vi "Create Database For Box IDs from cluster.vi"(8 "error in (no error)":errorcluster, 10 "Box ID Array":u8[](array[numeric])=[1, 2, 3, 4, 5, 6, 7, 8, 9, 10, 11, 12, 13, 14, 15], 11 "Calibration mode":bool) -> (0 "error out":errorcluster, 2 "Specific Frames":refnum<k21>[](array[refnum]), 3 "XNET Database out":refnum<k21>)   [LabVIEW 2021, in "BS120x Driver.lvlib" / "BS120x.lvclass"]
uses:
  BS120x.lvclass
  XNET Signal properties.ctl
  XNET Frame properties.ctl
  <vilib>/xnet/xnet.llb/XNET Database Create (Cluster).vi
  <vilib>/xnet/xnet.llb/XNET Database Create (Frame).vi
  <vilib>/xnet/xnet.llb/XNET Database Create (Signal).vi
  <resource>/objmgr/xnet.rc
panel:
  in  "Frames (Standard)":cluster{T1[], "XNET Frame properties":T2}[](array[cluster])=[{[{"ByteOrdr"=0, "Comment"="", "DataType"=1, "Default"=0.0, "Max"=5.0, "Min"=0.0, "NameShort"="AI_1", "NumBits"=16, "ScaleFac"=0.0001, "ScaleOff"=0.0, "StartBit"=0, "Unit"="V"}, {"ByteOrdr"=0, "Comment"="", "DataType"=1, "Default"=0.0, "Max"=5.0, "Min"=0.0, "NameShort"="AI_2", "NumBits"=16, "ScaleFac"=0.0001, "ScaleOff"=0.0, "StartBit"=16, "Unit"="V"}, {"ByteOrdr"=0, "Comment"="", "DataType"=1, "Default"=0.0, "Max"=5.0, "Min"=0.0, "NameShort"="AI_3", "NumBits"=16, "ScaleFac"=0.0001, "ScaleOff"=0.0, "StartBit"=32, "Unit"="V"}, {"ByteOrdr"=0, "Comment"="", "DataType"=1, "Default"=0.0, "Max"=5.0, "Min"=0.0, "NameShort"="AI_4", "NumBits"=16, "ScaleFac"=0.0001, "ScaleOff"=0.0, "StartBit"=48, "Unit"="V"}], "XNET Frame properties"={"NameShort"="AI_Readback_1_4", "ID"=672, "PayldLen"=8, "CAN.TimingType"=0, "CAN.TxTime"=0.01}}, {[{"ByteOrdr"=0, "Comment"="", "DataType"=1, "Default"=0.0, "Max"=5.0, "Min"=0.0, "NameShort"="AI_5", "NumBits"=16, "ScaleFac"=0.0001, "ScaleOff"=0.0, "StartBit"=0, "Unit"="V"}, {"ByteOrdr"=0, "Comment"="", "DataType"=1, "Default"=0.0, "Max"=5.0, "Min"=0.0, "NameShort"="AI_6", "NumBits"=16, "ScaleFac"=0.0001, "ScaleOff"=0.0, "StartBit"=16, "Unit"="V"}, {"ByteOrdr"=0, "Comment"="", "DataType"=1, "Default"=0.0, "Max"=5.0, "Min"=0.0, "NameShort"="AI_7", "NumBits"=16, "ScaleFac"=0.0001, "ScaleOff"=0.0, "StartBit"=32, "Unit"="V"}, {"ByteOrdr"=0, "Comment"="", "DataType"=1, "Default"=0.0, "Max"=5.0, "Min"=0.0, "NameShort"="AI_8", "NumBits"=16, "ScaleFac"=0.0001, "ScaleOff"=0.0, "StartBit"=48, "Unit"="V"}], "XNET Frame properties"={"NameShort"="AI_Readback_5_8", "ID"=688, "PayldLen"=8, "CAN.TimingType"=0, "CAN.TxTime"=0.01}}, {[{"ByteOrdr"=0, "Comment"="", "DataType"=1, "Default"=0.0, "Max"=5.0, "Min"=0.0, "NameShort"="AO1_Voltage", "NumBits"=16, "ScaleFac"=0.0001, "ScaleOff"=0.0, "StartBit"=0, "Unit"="V"}, {"ByteOrdr"=0, "Comment"="", "DataType"=1, "Default"=0.0, "Max"=5.0, "Min"=0.0, "NameShort"="AO2_Voltage", "NumBits"=16, "ScaleFac"=0.0001, "ScaleOff"=0.0, "StartBit"=16, "Unit"="V"}], "XNET Frame properties"={"NameShort"="Analog_Out_Set_1_2", "ID"=544, "PayldLen"=8, "CAN.TimingType"=1, "CAN.TxTime"=0.1}}, {[{"ByteOrdr"=0, "Comment"="", "DataType"=1, "Default"=1.0, "Max"=12.0, "Min"=1.0, "NameShort"="Channel", "NumBits"=8, "ScaleFac"=1.0, "ScaleOff"=1.0, "StartBit"=0, "Unit"=""}, {"ByteOrdr"=0, "Comment"="", "DataType"=1, "Default"=0.0, "Max"=1.0, "Min"=0.0, "NameShort"="Enable", "NumBits"=1, "ScaleFac"=1.0, "ScaleOff"=0.0, "StartBit"=8, "Unit"=""}], "XNET Frame properties"={"NameShort"="Cell_Enable", "ID"=1360, "PayldLen"=2, "CAN.TimingType"=1, "CAN.TxTime"=0.1}}, {[{"ByteOrdr"=0, "Comment"="", "DataType"=1, "Default"=0.0, "Max"=1.0, "Min"=0.0, "NameShort"="Enable", "NumBits"=1, "ScaleFac"=1.0, "ScaleOff"=0.0, "StartBit"=0, "Unit"=""}], "XNET Frame properties"={"NameShort"="Cell_Enable_All", "ID"=1344, "PayldLen"=1, "CAN.TimingType"=1, "CAN.TxTime"=0.1}}, {[{"ByteOrdr"=0, "Comment"="", "DataType"=1, "Default"=0.0, "Max"=500.0000000000003, "Min"=-500.0000000000003, "NameShort"="Cell_I_1", "NumBits"=16, "ScaleFac"=0.1, "ScaleOff"=-3276.800000000003, "StartBit"=0, "Unit"="mA"}, {"ByteOrdr"=0, "Comment"="", "DataType"=1, "Default"=0.0, "Max"=500.0000000000003, "Min"=-500.0000000000003, "NameShort"="Cell_I_2", "NumBits"=16, "ScaleFac"=0.1, "ScaleOff"=-3276.800000000003, "StartBit"=16, "Unit"="mA"}, {"ByteOrdr"=0, "Comment"="", "DataType"=1, "Default"=0.0, "Max"=500.0000000000003, "Min"=-500.0000000000003, "NameShort"="Cell_I_3", "NumBits"=16, "ScaleFac"=0.1, "ScaleOff"=-3276.800000000003, "StartBit"=32, "Unit"="mA"}, {"ByteOrdr"=0, "Comment"="", "DataType"=1, "Default"=0.0, "Max"=500.0000000000003, "Min"=-500.0000000000003, "NameShort"="Cell_I_4", "NumBits"=16, "ScaleFac"=0.1, "ScaleOff"=-3276.800000000003, "StartBit"=48, "Unit"="mA"}], "XNET Frame properties"={"NameShort"="Cell_I_Readback_1_4", "ID"=384, "PayldLen"=8, "CAN.TimingType"=0, "CAN.TxTime"=0.01}}, {[{"ByteOrdr"=0, "Comment"="", "DataType"=1, "Default"=0.0, "Max"=500.0000000000003, "Min"=-500.0000000000003, "NameShort"="Cell_I_5", "NumBits"=16, "ScaleFac"=0.1, "ScaleOff"=-3276.800000000003, "StartBit"=0, "Unit"="mA"}, {"ByteOrdr"=0, "Comment"="", "DataType"=1, "Default"=0.0, "Max"=500.0000000000003, "Min"=-500.0000000000003, "NameShort"="Cell_I_6", "NumBits"=16, "ScaleFac"=0.1, "ScaleOff"=-3276.800000000003, "StartBit"=16, "Unit"="mA"}, {"ByteOrdr"=0, "Comment"="", "DataType"=1, "Default"=0.0, "Max"=500.0000000000003, "Min"=-500.0000000000003, "NameShort"="Cell_I_7", "NumBits"=16, "ScaleFac"=0.1, "ScaleOff"=-3276.800000000003, "StartBit"=32, "Unit"="mA"}, {"ByteOrdr"=0, "Comment"="", "DataType"=1, "Default"=0.0, "Max"=500.0000000000003, "Min"=-500.0000000000003, "NameShort"="Cell_I_8", "NumBits"=16, "ScaleFac"=0.1, "ScaleOff"=-3276.800000000003, "StartBit"=48, "Unit"="mA"}], "XNET Frame properties"={"NameShort"="Cell_I_Readback_5_8", "ID"=400, "PayldLen"=8, "CAN.TimingType"=0, "CAN.TxTime"=0.01}}, {[{"ByteOrdr"=0, "Comment"="", "DataType"=1, "Default"=0.0, "Max"=500.0000000000003, "Min"=-500.0000000000003, "NameShort"="Cell_I_09", "NumBits"=16, "ScaleFac"=0.1, "ScaleOff"=-3276.800000000003, "StartBit"=0, "Unit"="mA"}, {"ByteOrdr"=0, "Comment"="", "DataType"=1, "Default"=0.0, "Max"=500.0000000000003, "Min"=-500.0000000000003, "NameShort"="Cell_I_10", "NumBits"=16, "ScaleFac"=0.1, "ScaleOff"=-3276.800000000003, "StartBit"=16, "Unit"="mA"}, {"ByteOrdr"=0, "Comment"="", "DataType"=1, "Default"=0.0, "Max"=500.0000000000003, "Min"=-500.0000000000003, "NameShort"="Cell_I_11", "NumBits"=16, "ScaleFac"=0.1, "ScaleOff"=-3276.800000000003, "StartBit"=32, "Unit"="mA"}, {"ByteOrdr"=0, "Comment"="", "DataType"=1, "Default"=0.0, "Max"=500.0000000000003, "Min"=-500.0000000000003, "NameShort"="Cell_I_12", "NumBits"=16, "ScaleFac"=0.1, "ScaleOff"=-3276.800000000003, "StartBit"=48, "Unit"="mA"}], "XNET Frame properties"={"NameShort"="Cell_I_Readback_9_12", "ID"=416, "PayldLen"=8, "CAN.TimingType"=0, "CAN.TxTime"=0.01}}, {[{"ByteOrdr"=0, "Comment"="", "DataType"=1, "Default"=0.0, "Max"=500.0000000000003, "Min"=-500.0000000000003, "NameShort"="Sink_I_All", "NumBits"=16, "ScaleFac"=0.1, "ScaleOff"=0.0, "StartBit"=16, "Unit"="mA"}, {"ByteOrdr"=0, "Comment"="", "DataType"=1, "Default"=0.0, "Max"=500.0000000000003, "Min"=-500.0000000000003, "NameShort"="Source_I_All", "NumBits"=16, "ScaleFac"=0.1, "ScaleOff"=0.0, "StartBit"=0, "Unit"="mA"}], "XNET Frame properties"={"NameShort"="Cell_I_Set_All", "ID"=1152, "PayldLen"=4, "CAN.TimingType"=1, "CAN.TxTime"=0.1}}, {[{"ByteOrdr"=0, "Comment"="", "DataType"=1, "Default"=1.0, "Max"=12.0, "Min"=1.0, "NameShort"="Channel", "NumBits"=8, "ScaleFac"=1.0, "ScaleOff"=1.0, "StartBit"=0, "Unit"=""}, {"ByteOrdr"=0, "Comment"="", "DataType"=1, "Default"=0.0, "Max"=500.0000000000003, "Min"=-500.0000000000003, "NameShort"="I_Sink", "NumBits"=16, "ScaleFac"=0.1, "ScaleOff"=0.0, "StartBit"=8, "Unit"="mA"}], "XNET Frame properties"={"NameShort"="Cell_I_Sink_Set", "ID"=1184, "PayldLen"=3, "CAN.TimingType"=1, "CAN.TxTime"=0.1}}, {[{"ByteOrdr"=0, "Comment"="", "DataType"=1, "Default"=1.0, "Max"=12.0, "Min"=1.0, "NameShort"="Channel", "NumBits"=8, "ScaleFac"=1.0, "ScaleOff"=1.0, "StartBit"=0, "Unit"=""}, {"ByteOrdr"=0, "Comment"="", "DataType"=1, "Default"=0.0, "Max"=500.0000000000003, "Min"=-500.0000000000003, "NameShort"="I_Source", "NumBits"=16, "ScaleFac"=0.1, "ScaleOff"=0.0, "StartBit"=8, "Unit"="mA"}], "XNET Frame properties"={"NameShort"="Cell_I_Source_Set", "ID"=1200, "PayldLen"=3, "CAN.TimingType"=1, "CAN.TxTime"=0.1}}, {[{"ByteOrdr"=0, "Comment"="", "DataType"=1, "Default"=0.0, "Max"=5.0, "Min"=0.0, "NameShort"="Cell_V_1", "NumBits"=16, "ScaleFac"=0.0001, "ScaleOff"=0.0, "StartBit"=0, "Unit"="V"}, {"ByteOrdr"=0, "Comment"="", "DataType"=1, "Default"=0.0, "Max"=5.0, "Min"=0.0, "NameShort"="Cell_V_2", "NumBits"=16, "ScaleFac"=0.0001, "ScaleOff"=0.0, "StartBit"=16, "Unit"="V"}, {"ByteOrdr"=0, "Comment"="", "DataType"=1, "Default"=0.0, "Max"=5.0, "Min"=0.0, "NameShort"="Cell_V_3", "NumBits"=16, "ScaleFac"=0.0001, "ScaleOff"=0.0, "StartBit"=32, "Unit"="V"}, {"ByteOrdr"=0, "Comment"="", "DataType"=1, "Default"=0.0, "Max"=5.0, "Min"=0.0, "NameShort"="Cell_V_4", "NumBits"=16, "ScaleFac"=0.0001, "ScaleOff"=0.0, "StartBit"=48, "Unit"="V"}], "XNET Frame properties"={"NameShort"="Cell_V_Readback_1_4", "ID"=288, "PayldLen"=8, "CAN.TimingType"=0, "CAN.TxTime"=0.01}}, {[{"ByteOrdr"=0, "Comment"="", "DataType"=1, "Default"=0.0, "Max"=5.0, "Min"=0.0, "NameShort"="Cell_V_5", "NumBits"=16, "ScaleFac"=0.0001, "ScaleOff"=0.0, "StartBit"=0, "Unit"="V"}, {"ByteOrdr"=0, "Comment"="", "DataType"=1, "Default"=0.0, "Max"=5.0, "Min"=0.0, "NameShort"="Cell_V_6", "NumBits"=16, "ScaleFac"=0.0001, "ScaleOff"=0.0, "StartBit"=16, "Unit"="V"}, {"ByteOrdr"=0, "Comment"="", "DataType"=1, "Default"=0.0, "Max"=5.0, "Min"=0.0, "NameShort"="Cell_V_7", "NumBits"=16, "ScaleFac"=0.0001, "ScaleOff"=0.0, "StartBit"=32, "Unit"="V"}, {"ByteOrdr"=0, "Comment"="", "DataType"=1, "Default"=0.0, "Max"=5.0, "Min"=0.0, "NameShort"="Cell_V_8", "NumBits"=16, "ScaleFac"=0.0001, "ScaleOff"=0.0, "StartBit"=48, "Unit"="V"}], "XNET Frame properties"={"NameShort"="Cell_V_Readback_5_8", "ID"=304, "PayldLen"=8, "CAN.TimingType"=0, "CAN.TxTime"=0.01}}, {[{"ByteOrdr"=0, "Comment"="", "DataType"=1, "Default"=0.0, "Max"=5.0, "Min"=0.0, "NameShort"="Cell_V_09", "NumBits"=16, "ScaleFac"=0.0001, "ScaleOff"=0.0, "StartBit"=0, "Unit"="V"}, {"ByteOrdr"=0, "Comment"="", "DataType"=1, "Default"=0.0, "Max"=5.0, "Min"=0.0, "NameShort"="Cell_V_10", "NumBits"=16, "ScaleFac"=0.0001, "ScaleOff"=0.0, "StartBit"=16, "Unit"="V"}, {"ByteOrdr"=0, "Comment"="", "DataType"=1, "Default"=0.0, "Max"=5.0, "Min"=0.0, "NameShort"="Cell_V_11", "NumBits"=16, "ScaleFac"=0.0001, "ScaleOff"=0.0, "StartBit"=32, "Unit"="V"}, {"ByteOrdr"=0, "Comment"="", "DataType"=1, "Default"=0.0, "Max"=5.0, "Min"=0.0, "NameShort"="Cell_V_12", "NumBits"=16, "ScaleFac"=0.0001, "ScaleOff"=0.0, "StartBit"=48, "Unit"="V"}], "XNET Frame properties"={"NameShort"="Cell_V_Readback_9_12", "ID"=320, "PayldLen"=8, "CAN.TimingType"=0, "CAN.TxTime"=0.01}}, {[{"ByteOrdr"=0, "Comment"="", "DataType"=1, "Default"=0.0, "Max"=5.0, "Min"=0.0, "NameShort"="Cell_Voltage", "NumBits"=16, "ScaleFac"=0.0001, "ScaleOff"=0.0, "StartBit"=8, "Unit"="V"}, {"ByteOrdr"=0, "Comment"="", "DataType"=1, "Default"=1.0, "Max"=12.0, "Min"=1.0, "NameShort"="Channel", "NumBits"=8, "ScaleFac"=1.0, "ScaleOff"=1.0, "StartBit"=0, "Unit"=""}], "XNET Frame properties"={"NameShort"="Cell_V_Set", "ID"=1296, "PayldLen"=3, "CAN.TimingType"=1, "CAN.TxTime"=0.1}}, {[{"ByteOrdr"=0, "Comment"="", "DataType"=1, "Default"=0.0, "Max"=5.0, "Min"=0.0, "NameShort"="Cell_1_Voltage", "NumBits"=16, "ScaleFac"=0.0001, "ScaleOff"=0.0, "StartBit"=0, "Unit"="V"}, {"ByteOrdr"=0, "Comment"="", "DataType"=1, "Default"=0.0, "Max"=5.0, "Min"=0.0, "NameShort"="Cell_2_Voltage", "NumBits"=16, "ScaleFac"=0.0001, "ScaleOff"=0.0, "StartBit"=16, "Unit"="V"}, {"ByteOrdr"=0, "Comment"="", "DataType"=1, "Default"=0.0, "Max"=5.0, "Min"=0.0, "NameShort"="Cell_3_Voltage", "NumBits"=16, "ScaleFac"=0.0001, "ScaleOff"=0.0, "StartBit"=32, "Unit"="V"}, {"ByteOrdr"=0, "Comment"="", "DataType"=1, "Default"=0.0, "Max"=5.0, "Min"=0.0, "NameShort"="Cell_4_Voltage", "NumBits"=16, "ScaleFac"=0.0001, "ScaleOff"=0.0, "StartBit"=48, "Unit"=""}], "XNET Frame properties"={"NameShort"="Cell_V_Set_1_4", "ID"=160, "PayldLen"=8, "CAN.TimingType"=1, "CAN.TxTime"=0.1}}, {[{"ByteOrdr"=0, "Comment"="", "DataType"=1, "Default"=0.0, "Max"=5.0, "Min"=0.0, "NameShort"="Cell_5_Voltage", "NumBits"=16, "ScaleFac"=0.0001, "ScaleOff"=0.0, "StartBit"=0, "Unit"="V"}, {"ByteOrdr"=0, "Comment"="", "DataType"=1, "Default"=0.0, "Max"=5.0, "Min"=0.0, "NameShort"="Cell_6_Voltage", "NumBits"=16, "ScaleFac"=0.0001, "ScaleOff"=0.0, "StartBit"=16, "Unit"="V"}, {"ByteOrdr"=0, "Comment"="", "DataType"=1, "Default"=0.0, "Max"=5.0, "Min"=0.0, "NameShort"="Cell_7_Voltage", "NumBits"=16, "ScaleFac"=0.0001, "ScaleOff"=0.0, "StartBit"=32, "Unit"="V"}, {"ByteOrdr"=0, "Comment"="", "DataType"=1, "Default"=0.0, "Max"=5.0, "Min"=0.0, "NameShort"="Cell_8_Voltage", "NumBits"=16, "ScaleFac"=0.0001, "ScaleOff"=0.0, "StartBit"=48, "Unit"="V"}], "XNET Frame properties"={"NameShort"="Cell_V_Set_5_8", "ID"=176, "PayldLen"=8, "CAN.TimingType"=1, "CAN.TxTime"=0.1}}, {[{"ByteOrdr"=0, "Comment"="", "DataType"=1, "Default"=0.0, "Max"=5.0, "Min"=0.0, "NameShort"="Cell_Voltage_10", "NumBits"=16, "ScaleFac"=0.0001, "ScaleOff"=0.0, "StartBit"=16, "Unit"="V"}, {"ByteOrdr"=0, "Comment"="", "DataType"=1, "Default"=0.0, "Max"=5.0, "Min"=0.0, "NameShort"="Cell_Voltage_11", "NumBits"=16, "ScaleFac"=0.0001, "ScaleOff"=0.0, "StartBit"=32, "Unit"="V"}, {"ByteOrdr"=0, "Comment"="", "DataType"=1, "Default"=0.0, "Max"=5.0, "Min"=0.0, "NameShort"="Cell_Voltage_12", "NumBits"=16, "ScaleFac"=0.0001, "ScaleOff"=0.0, "StartBit"=48, "Unit"="V"}, {"ByteOrdr"=0, "Comment"="", "DataType"=1, "Default"=0.0, "Max"=5.0, "Min"=0.0, "NameShort"="Cell_Voltage_9", "NumBits"=16, "ScaleFac"=0.0001, "ScaleOff"=0.0, "StartBit"=0, "Unit"="V"}], "XNET Frame properties"={"NameShort"="Cell_V_Set_9_12", "ID"=192, "PayldLen"=8, "CAN.TimingType"=1, "CAN.TxTime"=0.1}}, {[{"ByteOrdr"=0, "Comment"="", "DataType"=1, "Default"=0.0, "Max"=5.0, "Min"=0.0, "NameShort"="Cell_Voltage_All", "NumBits"=16, "ScaleFac"=0.0001, "ScaleOff"=0.0, "StartBit"=0, "Unit"="V"}], "XNET Frame properties"={"NameShort"="Cell_V_Set_All", "ID"=1280, "PayldLen"=2, "CAN.TimingType"=1, "CAN.TxTime"=0.1}}, {[{"ByteOrdr"=0, "Comment"="", "DataType"=1, "Default"=0.0, "Max"=1.0, "Min"=0.0, "NameShort"="AI_1_4_HIL_BCast_Enable", "NumBits"=1, "ScaleFac"=1.0, "ScaleOff"=0.0, "StartBit"=9, "Unit"=""}, {"ByteOrdr"=0, "Comment"="", "DataType"=1, "Default"=0.0, "Max"=1.0, "Min"=0.0, "NameShort"="AI_5_8_HIL_BCast_Enable", "NumBits"=1, "ScaleFac"=1.0, "ScaleOff"=0.0, "StartBit"=10, "Unit"=""}, {"ByteOrdr"=0, "Comment"="", "DataType"=1, "Default"=0.0, "Max"=1.0, "Min"=0.0, "NameShort"="AO_HIL_Set_Enable", "NumBits"=1, "ScaleFac"=1.0, "ScaleOff"=0.0, "StartBit"=1, "Unit"=""}, {"ByteOrdr"=0, "Comment"="", "DataType"=1, "Default"=0.0, "Max"=1000.0, "Min"=0.0, "NameShort"="Calibration_Mode", "NumBits"=1, "ScaleFac"=1.0, "ScaleOff"=0.0, "StartBit"=16, "Unit"=""}, {"ByteOrdr"=0, "Comment"="", "DataType"=1, "Default"=0.0, "Max"=1.0, "Min"=0.0, "NameShort"="DIO_HIL_BCast_Enable", "NumBits"=1, "ScaleFac"=1.0, "ScaleOff"=0.0, "StartBit"=8, "Unit"=""}, {"ByteOrdr"=0, "Comment"="", "DataType"=1, "Default"=0.0, "Max"=1.0, "Min"=0.0, "NameShort"="DIO_HIL_Set_Enable", "NumBits"=1, "ScaleFac"=1.0, "ScaleOff"=0.0, "StartBit"=0, "Unit"=""}], "XNET Frame properties"={"NameShort"="Configure", "ID"=1024, "PayldLen"=3, "CAN.TimingType"=1, "CAN.TxTime"=0.1}}, {[{"ByteOrdr"=0, "Comment"="", "DataType"=1, "Default"=0.0, "Max"=1.0, "Min"=0.0, "NameShort"="Calibration_Enable", "NumBits"=1, "ScaleFac"=1.0, "ScaleOff"=0.0, "StartBit"=0, "Unit"=""}, {"ByteOrdr"=1, "Comment"="", "DataType"=1, "Default"=0.0, "Max"=1.0, "Min"=0.0, "NameShort"="PID_Disable", "NumBits"=1, "ScaleFac"=1.0, "ScaleOff"=0.0, "StartBit"=1, "Unit"=""}, {"ByteOrdr"=2, "Comment"="", "DataType"=1, "Default"=0.0, "Max"=1.0, "Min"=0.0, "NameShort"="Precision_Mode_Enable", "NumBits"=1, "ScaleFac"=1.0, "ScaleOff"=0.0, "StartBit"=8, "Unit"=""}], "XNET Frame properties"={"NameShort"="OperationalConfig", "ID"=1040, "PayldLen"=2, "CAN.TimingType"=1, "CAN.TxTime"=0.1}}, {[{"ByteOrdr"=0, "Comment"="", "DataType"=1, "Default"=0.0, "Max"=255.0, "Min"=0.0, "NameShort"="DIO_1_8", "NumBits"=8, "ScaleFac"=1.0, "ScaleOff"=0.0, "StartBit"=0, "Unit"=""}], "XNET Frame properties"={"NameShort"="DIO_Readback_1_8", "ID"=640, "PayldLen"=8, "CAN.TimingType"=0, "CAN.TxTime"=0.01}}, {[{"ByteOrdr"=0, "Comment"="", "DataType"=1, "Default"=0.0, "Max"=255.0, "Min"=0.0, "NameShort"="DIO_Direction", "NumBits"=8, "ScaleFac"=1.0, "ScaleOff"=0.0, "StartBit"=8, "Unit"=""}, {"ByteOrdr"=0, "Comment"="", "DataType"=1, "Default"=0.0, "Max"=255.0, "Min"=0.0, "NameShort"="DIO_Output_Val", "NumBits"=8, "ScaleFac"=1.0, "ScaleOff"=0.0, "StartBit"=0, "Unit"=""}], "XNET Frame properties"={"NameShort"="Digital_IO_Set_1_8", "ID"=512, "PayldLen"=2, "CAN.TimingType"=1, "CAN.TxTime"=0.1}}, {[{"ByteOrdr"=0, "Comment"="Set to True to enable HIL mode", "DataType"=1, "Default"=0.0, "Max"=1000.0, "Min"=0.0, "NameShort"="Enable", "NumBits"=1, "ScaleFac"=1.0, "ScaleOff"=0.0, "StartBit"=0, "Unit"=""}], "XNET Frame properties"={"NameShort"="HIL_Mode", "ID"=128, "PayldLen"=1, "CAN.TimingType"=1, "CAN.TxTime"=0.1}}, {[{"ByteOrdr"=0, "Comment"="", "DataType"=1, "Default"=0.0, "Max"=1.0, "Min"=0.0, "NameShort"="Fan_Fail_1", "NumBits"=1, "ScaleFac"=1.0, "ScaleOff"=0.0, "StartBit"=0, "Unit"=""}, {"ByteOrdr"=0, "Comment"="", "DataType"=1, "Default"=0.0, "Max"=1.0, "Min"=0.0, "NameShort"="Fan_Fail_2", "NumBits"=1, "ScaleFac"=1.0, "ScaleOff"=0.0, "StartBit"=1, "Unit"=""}, {"ByteOrdr"=0, "Comment"="", "DataType"=1, "Default"=0.0, "Max"=1.0, "Min"=0.0, "NameShort"="Fan_Fail_3", "NumBits"=1, "ScaleFac"=1.0, "ScaleOff"=0.0, "StartBit"=2, "Unit"=""}, {"ByteOrdr"=0, "Comment"="", "DataType"=1, "Default"=0.0, "Max"=1.0, "Min"=0.0, "NameShort"="Fan_Fail_4", "NumBits"=1, "ScaleFac"=1.0, "ScaleOff"=0.0, "StartBit"=3, "Unit"=""}, {"ByteOrdr"=0, "Comment"="", "DataType"=1, "Default"=0.0, "Max"=1.0, "Min"=0.0, "NameShort"="Inhibit_State", "NumBits"=1, "ScaleFac"=1.0, "ScaleOff"=0.0, "StartBit"=4, "Unit"=""}, {"ByteOrdr"=0, "Comment"="", "DataType"=1, "Default"=0.0, "Max"=1000.0, "Min"=0.0, "NameShort"="Temp_Sensor_1", "NumBits"=8, "ScaleFac"=1.0, "ScaleOff"=0.0, "StartBit"=8, "Unit"="Degrees C"}, {"ByteOrdr"=0, "Comment"="", "DataType"=1, "Default"=0.0, "Max"=1000.0, "Min"=0.0, "NameShort"="Temp_Sensor_2", "NumBits"=8, "ScaleFac"=1.0, "ScaleOff"=0.0, "StartBit"=16, "Unit"="Degrees C"}, {"ByteOrdr"=0, "Comment"="", "DataType"=1, "Default"=0.0, "Max"=1000.0, "Min"=0.0, "NameShort"="Temp_Sensor_3", "NumBits"=8, "ScaleFac"=1.0, "ScaleOff"=0.0, "StartBit"=24, "Unit"="Degrees C"}], "XNET Frame properties"={"NameShort"="System_Status", "ID"=256, "PayldLen"=8, "CAN.TimingType"=0, "CAN.TxTime"=1.0}}] {"XNET Frame properties"."ID" format="%.0x"}
  in  "Database Cluster":string="BS1200_Control_Bus"
  in  "Frames (Calibration)":cluster{T1[], "XNET Frame properties":T2}[](array[cluster])=[{[{"ByteOrdr"=0, "Comment"="", "DataType"=1, "Default"=0.0, "Max"=5.0, "Min"=0.0, "NameShort"="AI_1", "NumBits"=16, "ScaleFac"=1.0, "ScaleOff"=0.0, "StartBit"=0, "Unit"="V"}, {"ByteOrdr"=0, "Comment"="", "DataType"=1, "Default"=0.0, "Max"=5.0, "Min"=0.0, "NameShort"="AI_2", "NumBits"=16, "ScaleFac"=1.0, "ScaleOff"=0.0, "StartBit"=16, "Unit"="V"}, {"ByteOrdr"=0, "Comment"="", "DataType"=1, "Default"=0.0, "Max"=5.0, "Min"=0.0, "NameShort"="AI_3", "NumBits"=16, "ScaleFac"=1.0, "ScaleOff"=0.0, "StartBit"=32, "Unit"="V"}, {"ByteOrdr"=0, "Comment"="", "DataType"=1, "Default"=0.0, "Max"=5.0, "Min"=0.0, "NameShort"="AI_4", "NumBits"=16, "ScaleFac"=1.0, "ScaleOff"=0.0, "StartBit"=48, "Unit"="V"}], "XNET Frame properties"={"NameShort"="AI_Readback_1_4", "ID"=672, "PayldLen"=8, "CAN.TimingType"=0, "CAN.TxTime"=0.01}}, {[{"ByteOrdr"=0, "Comment"="", "DataType"=1, "Default"=0.0, "Max"=1000.0, "Min"=0.0, "NameShort"="AI_5", "NumBits"=16, "ScaleFac"=1.0, "ScaleOff"=0.0, "StartBit"=0, "Unit"="V"}, {"ByteOrdr"=0, "Comment"="", "DataType"=1, "Default"=0.0, "Max"=5.0, "Min"=0.0, "NameShort"="AI_6", "NumBits"=16, "ScaleFac"=1.0, "ScaleOff"=0.0, "StartBit"=16, "Unit"="V"}, {"ByteOrdr"=0, "Comment"="", "DataType"=1, "Default"=0.0, "Max"=5.0, "Min"=0.0, "NameShort"="AI_7", "NumBits"=16, "ScaleFac"=1.0, "ScaleOff"=0.0, "StartBit"=32, "Unit"="V"}, {"ByteOrdr"=0, "Comment"="", "DataType"=1, "Default"=0.0, "Max"=5.0, "Min"=0.0, "NameShort"="AI_8", "NumBits"=16, "ScaleFac"=1.0, "ScaleOff"=0.0, "StartBit"=48, "Unit"="V"}], "XNET Frame properties"={"NameShort"="AI_Readback_5_8", "ID"=688, "PayldLen"=8, "CAN.TimingType"=0, "CAN.TxTime"=0.01}}, {[{"ByteOrdr"=0, "Comment"="", "DataType"=1, "Default"=0.0, "Max"=5.0, "Min"=0.0, "NameShort"="AO1_Voltage", "NumBits"=16, "ScaleFac"=1.0, "ScaleOff"=0.0, "StartBit"=0, "Unit"="V"}, {"ByteOrdr"=0, "Comment"="", "DataType"=1, "Default"=0.0, "Max"=5.0, "Min"=0.0, "NameShort"="AO2_Voltage", "NumBits"=16, "ScaleFac"=1.0, "ScaleOff"=0.0, "StartBit"=16, "Unit"="V"}], "XNET Frame properties"={"NameShort"="Analog_Out_Set_1_2", "ID"=544, "PayldLen"=8, "CAN.TimingType"=1, "CAN.TxTime"=0.1}}, {[{"ByteOrdr"=0, "Comment"="", "DataType"=1, "Default"=1.0, "Max"=12.0, "Min"=1.0, "NameShort"="Channel", "NumBits"=8, "ScaleFac"=1.0, "ScaleOff"=1.0, "StartBit"=0, "Unit"=""}, {"ByteOrdr"=0, "Comment"="", "DataType"=1, "Default"=0.0, "Max"=1.0, "Min"=0.0, "NameShort"="Enable", "NumBits"=1, "ScaleFac"=1.0, "ScaleOff"=0.0, "StartBit"=8, "Unit"=""}], "XNET Frame properties"={"NameShort"="Cell_Enable", "ID"=1360, "PayldLen"=2, "CAN.TimingType"=1, "CAN.TxTime"=0.1}}, {[{"ByteOrdr"=0, "Comment"="", "DataType"=1, "Default"=0.0, "Max"=1.0, "Min"=0.0, "NameShort"="Enable", "NumBits"=1, "ScaleFac"=1.0, "ScaleOff"=0.0, "StartBit"=0, "Unit"=""}], "XNET Frame properties"={"NameShort"="Cell_Enable_All", "ID"=1344, "PayldLen"=1, "CAN.TimingType"=1, "CAN.TxTime"=0.1}}, {[{"ByteOrdr"=0, "Comment"="", "DataType"=1, "Default"=0.0, "Max"=500.0000000000002, "Min"=-500.0000000000002, "NameShort"="Cell_I_1", "NumBits"=16, "ScaleFac"=1.0, "ScaleOff"=0.0, "StartBit"=0, "Unit"="mA"}, {"ByteOrdr"=0, "Comment"="", "DataType"=1, "Default"=0.0, "Max"=500.0000000000002, "Min"=-500.0000000000002, "NameShort"="Cell_I_2", "NumBits"=16, "ScaleFac"=1.0, "ScaleOff"=0.0, "StartBit"=16, "Unit"="mA"}, {"ByteOrdr"=0, "Comment"="", "DataType"=1, "Default"=0.0, "Max"=500.0000000000002, "Min"=-500.0000000000002, "NameShort"="Cell_I_3", "NumBits"=16, "ScaleFac"=1.0, "ScaleOff"=0.0, "StartBit"=32, "Unit"="mA"}, {"ByteOrdr"=0, "Comment"="", "DataType"=1, "Default"=0.0, "Max"=500.0000000000002, "Min"=-500.0000000000002, "NameShort"="Cell_I_4", "NumBits"=16, "ScaleFac"=1.0, "ScaleOff"=0.0, "StartBit"=48, "Unit"="mA"}], "XNET Frame properties"={"NameShort"="Cell_I_Readback_1_4", "ID"=384, "PayldLen"=8, "CAN.TimingType"=0, "CAN.TxTime"=0.01}}, {[{"ByteOrdr"=0, "Comment"="", "DataType"=1, "Default"=0.0, "Max"=500.0000000000002, "Min"=-500.0000000000002, "NameShort"="Cell_I_5", "NumBits"=16, "ScaleFac"=1.0, "ScaleOff"=0.0, "StartBit"=0, "Unit"="mA"}, {"ByteOrdr"=0, "Comment"="", "DataType"=1, "Default"=0.0, "Max"=500.0000000000002, "Min"=-500.0000000000002, "NameShort"="Cell_I_6", "NumBits"=16, "ScaleFac"=1.0, "ScaleOff"=0.0, "StartBit"=16, "Unit"="mA"}, {"ByteOrdr"=0, "Comment"="", "DataType"=1, "Default"=0.0, "Max"=500.0000000000002, "Min"=-500.0000000000002, "NameShort"="Cell_I_7", "NumBits"=16, "ScaleFac"=1.0, "ScaleOff"=0.0, "StartBit"=32, "Unit"="mA"}, {"ByteOrdr"=0, "Comment"="", "DataType"=1, "Default"=0.0, "Max"=500.0000000000002, "Min"=-500.0000000000002, "NameShort"="Cell_I_8", "NumBits"=16, "ScaleFac"=1.0, "ScaleOff"=0.0, "StartBit"=48, "Unit"="mA"}], "XNET Frame properties"={"NameShort"="Cell_I_Readback_5_8", "ID"=400, "PayldLen"=8, "CAN.TimingType"=0, "CAN.TxTime"=0.01}}, {[{"ByteOrdr"=0, "Comment"="", "DataType"=1, "Default"=0.0, "Max"=500.0000000000002, "Min"=-500.0000000000002, "NameShort"="Cell_I_09", "NumBits"=16, "ScaleFac"=1.0, "ScaleOff"=0.0, "StartBit"=0, "Unit"="mA"}, {"ByteOrdr"=0, "Comment"="", "DataType"=1, "Default"=0.0, "Max"=500.0000000000002, "Min"=-500.0000000000002, "NameShort"="Cell_I_10", "NumBits"=16, "ScaleFac"=1.0, "ScaleOff"=0.0, "StartBit"=16, "Unit"="mA"}, {"ByteOrdr"=0, "Comment"="", "DataType"=1, "Default"=0.0, "Max"=500.0000000000002, "Min"=-500.0000000000002, "NameShort"="Cell_I_11", "NumBits"=16, "ScaleFac"=1.0, "ScaleOff"=0.0, "StartBit"=32, "Unit"="mA"}, {"ByteOrdr"=0, "Comment"="", "DataType"=1, "Default"=0.0, "Max"=500.0000000000002, "Min"=-500.0000000000002, "NameShort"="Cell_I_12", "NumBits"=16, "ScaleFac"=1.0, "ScaleOff"=0.0, "StartBit"=48, "Unit"="mA"}], "XNET Frame properties"={"NameShort"="Cell_I_Readback_9_12", "ID"=416, "PayldLen"=8, "CAN.TimingType"=0, "CAN.TxTime"=0.01}}, {[{"ByteOrdr"=0, "Comment"="", "DataType"=1, "Default"=0.0, "Max"=500.0000000000002, "Min"=0.0, "NameShort"="Sink_I_All", "NumBits"=16, "ScaleFac"=1.0, "ScaleOff"=0.0, "StartBit"=16, "Unit"="mA"}, {"ByteOrdr"=0, "Comment"="", "DataType"=1, "Default"=0.0, "Max"=500.0000000000002, "Min"=0.0, "NameShort"="Source_I_All", "NumBits"=16, "ScaleFac"=1.0, "ScaleOff"=0.0, "StartBit"=0, "Unit"="mA"}], "XNET Frame properties"={"NameShort"="Cell_I_Set_All", "ID"=1152, "PayldLen"=4, "CAN.TimingType"=1, "CAN.TxTime"=0.1}}, {[{"ByteOrdr"=0, "Comment"="", "DataType"=1, "Default"=1.0, "Max"=12.0, "Min"=1.0, "NameShort"="Channel", "NumBits"=8, "ScaleFac"=1.0, "ScaleOff"=1.0, "StartBit"=0, "Unit"=""}, {"ByteOrdr"=0, "Comment"="", "DataType"=1, "Default"=0.0, "Max"=500.0000000000002, "Min"=0.0, "NameShort"="I_Sink", "NumBits"=16, "ScaleFac"=1.0, "ScaleOff"=0.0, "StartBit"=8, "Unit"="mA"}], "XNET Frame properties"={"NameShort"="Cell_I_Sink_Set", "ID"=1184, "PayldLen"=3, "CAN.TimingType"=1, "CAN.TxTime"=0.1}}, {[{"ByteOrdr"=0, "Comment"="", "DataType"=1, "Default"=1.0, "Max"=12.0, "Min"=1.0, "NameShort"="Channel", "NumBits"=8, "ScaleFac"=1.0, "ScaleOff"=1.0, "StartBit"=0, "Unit"=""}, {"ByteOrdr"=0, "Comment"="", "DataType"=1, "Default"=0.0, "Max"=500.0000000000002, "Min"=0.0, "NameShort"="I_Source", "NumBits"=16, "ScaleFac"=1.0, "ScaleOff"=0.0, "StartBit"=8, "Unit"="mA"}], "XNET Frame properties"={"NameShort"="Cell_I_Source_Set", "ID"=1200, "PayldLen"=3, "CAN.TimingType"=1, "CAN.TxTime"=0.1}}, {[{"ByteOrdr"=0, "Comment"="", "DataType"=1, "Default"=0.0, "Max"=5.0, "Min"=0.0, "NameShort"="Cell_V_1", "NumBits"=16, "ScaleFac"=1.0, "ScaleOff"=0.0, "StartBit"=0, "Unit"="V"}, {"ByteOrdr"=0, "Comment"="", "DataType"=1, "Default"=0.0, "Max"=5.0, "Min"=0.0, "NameShort"="Cell_V_2", "NumBits"=16, "ScaleFac"=1.0, "ScaleOff"=0.0, "StartBit"=16, "Unit"="V"}, {"ByteOrdr"=0, "Comment"="", "DataType"=1, "Default"=0.0, "Max"=5.0, "Min"=0.0, "NameShort"="Cell_V_3", "NumBits"=16, "ScaleFac"=1.0, "ScaleOff"=0.0, "StartBit"=32, "Unit"="V"}, {"ByteOrdr"=0, "Comment"="", "DataType"=1, "Default"=0.0, "Max"=5.0, "Min"=0.0, "NameShort"="Cell_V_4", "NumBits"=16, "ScaleFac"=1.0, "ScaleOff"=0.0, "StartBit"=48, "Unit"="V"}], "XNET Frame properties"={"NameShort"="Cell_V_Readback_1_4", "ID"=288, "PayldLen"=8, "CAN.TimingType"=0, "CAN.TxTime"=0.01}}, {[{"ByteOrdr"=0, "Comment"="", "DataType"=1, "Default"=0.0, "Max"=5.0, "Min"=0.0, "NameShort"="Cell_V_5", "NumBits"=16, "ScaleFac"=1.0, "ScaleOff"=0.0, "StartBit"=0, "Unit"="V"}, {"ByteOrdr"=0, "Comment"="", "DataType"=1, "Default"=0.0, "Max"=5.0, "Min"=0.0, "NameShort"="Cell_V_6", "NumBits"=16, "ScaleFac"=1.0, "ScaleOff"=0.0, "StartBit"=16, "Unit"="V"}, {"ByteOrdr"=0, "Comment"="", "DataType"=1, "Default"=0.0, "Max"=5.0, "Min"=0.0, "NameShort"="Cell_V_7", "NumBits"=16, "ScaleFac"=1.0, "ScaleOff"=0.0, "StartBit"=32, "Unit"="V"}, {"ByteOrdr"=0, "Comment"="", "DataType"=1, "Default"=0.0, "Max"=5.0, "Min"=0.0, "NameShort"="Cell_V_8", "NumBits"=16, "ScaleFac"=1.0, "ScaleOff"=0.0, "StartBit"=48, "Unit"="V"}], "XNET Frame properties"={"NameShort"="Cell_V_Readback_5_8", "ID"=304, "PayldLen"=8, "CAN.TimingType"=0, "CAN.TxTime"=0.01}}, {[{"ByteOrdr"=0, "Comment"="", "DataType"=1, "Default"=0.0, "Max"=5.0, "Min"=0.0, "NameShort"="Cell_V_09", "NumBits"=16, "ScaleFac"=1.0, "ScaleOff"=0.0, "StartBit"=0, "Unit"="V"}, {"ByteOrdr"=0, "Comment"="", "DataType"=1, "Default"=0.0, "Max"=5.0, "Min"=0.0, "NameShort"="Cell_V_10", "NumBits"=16, "ScaleFac"=1.0, "ScaleOff"=0.0, "StartBit"=16, "Unit"="V"}, {"ByteOrdr"=0, "Comment"="", "DataType"=1, "Default"=0.0, "Max"=5.0, "Min"=0.0, "NameShort"="Cell_V_11", "NumBits"=16, "ScaleFac"=1.0, "ScaleOff"=0.0, "StartBit"=32, "Unit"="V"}, {"ByteOrdr"=0, "Comment"="", "DataType"=1, "Default"=0.0, "Max"=5.0, "Min"=0.0, "NameShort"="Cell_V_12", "NumBits"=16, "ScaleFac"=1.0, "ScaleOff"=0.0, "StartBit"=48, "Unit"="V"}], "XNET Frame properties"={"NameShort"="Cell_V_Readback_9_12", "ID"=320, "PayldLen"=8, "CAN.TimingType"=0, "CAN.TxTime"=0.01}}, {[{"ByteOrdr"=0, "Comment"="", "DataType"=1, "Default"=0.0, "Max"=5.0, "Min"=0.0, "NameShort"="Cell_Voltage", "NumBits"=16, "ScaleFac"=1.0, "ScaleOff"=0.0, "StartBit"=8, "Unit"="V"}, {"ByteOrdr"=0, "Comment"="", "DataType"=1, "Default"=1.0, "Max"=12.0, "Min"=1.0, "NameShort"="Channel", "NumBits"=8, "ScaleFac"=1.0, "ScaleOff"=1.0, "StartBit"=0, "Unit"=""}], "XNET Frame properties"={"NameShort"="Cell_V_Set", "ID"=1296, "PayldLen"=3, "CAN.TimingType"=1, "CAN.TxTime"=0.1}}, {[{"ByteOrdr"=0, "Comment"="", "DataType"=1, "Default"=0.0, "Max"=5.0, "Min"=0.0, "NameShort"="Cell_1_Voltage", "NumBits"=16, "ScaleFac"=1.0, "ScaleOff"=0.0, "StartBit"=0, "Unit"="V"}, {"ByteOrdr"=0, "Comment"="", "DataType"=1, "Default"=0.0, "Max"=5.0, "Min"=0.0, "NameShort"="Cell_2_Voltage", "NumBits"=16, "ScaleFac"=1.0, "ScaleOff"=0.0, "StartBit"=16, "Unit"="V"}, {"ByteOrdr"=0, "Comment"="", "DataType"=1, "Default"=0.0, "Max"=5.0, "Min"=0.0, "NameShort"="Cell_3_Voltage", "NumBits"=16, "ScaleFac"=1.0, "ScaleOff"=0.0, "StartBit"=32, "Unit"="V"}, {"ByteOrdr"=0, "Comment"="", "DataType"=1, "Default"=0.0, "Max"=5.0, "Min"=0.0, "NameShort"="Cell_4_Voltage", "NumBits"=16, "ScaleFac"=1.0, "ScaleOff"=0.0, "StartBit"=48, "Unit"=""}], "XNET Frame properties"={"NameShort"="Cell_V_Set_1_4", "ID"=160, "PayldLen"=8, "CAN.TimingType"=1, "CAN.TxTime"=0.1}}, {[{"ByteOrdr"=0, "Comment"="", "DataType"=1, "Default"=0.0, "Max"=5.0, "Min"=0.0, "NameShort"="Cell_5_Voltage", "NumBits"=16, "ScaleFac"=1.0, "ScaleOff"=0.0, "StartBit"=0, "Unit"="V"}, {"ByteOrdr"=0, "Comment"="", "DataType"=1, "Default"=0.0, "Max"=5.0, "Min"=0.0, "NameShort"="Cell_6_Voltage", "NumBits"=16, "ScaleFac"=1.0, "ScaleOff"=0.0, "StartBit"=16, "Unit"="V"}, {"ByteOrdr"=0, "Comment"="", "DataType"=1, "Default"=0.0, "Max"=5.0, "Min"=0.0, "NameShort"="Cell_7_Voltage", "NumBits"=16, "ScaleFac"=1.0, "ScaleOff"=0.0, "StartBit"=32, "Unit"="V"}, {"ByteOrdr"=0, "Comment"="", "DataType"=1, "Default"=0.0, "Max"=5.0, "Min"=0.0, "NameShort"="Cell_8_Voltage", "NumBits"=16, "ScaleFac"=1.0, "ScaleOff"=0.0, "StartBit"=48, "Unit"="V"}], "XNET Frame properties"={"NameShort"="Cell_V_Set_5_8", "ID"=176, "PayldLen"=8, "CAN.TimingType"=1, "CAN.TxTime"=0.1}}, {[{"ByteOrdr"=0, "Comment"="", "DataType"=1, "Default"=0.0, "Max"=5.0, "Min"=0.0, "NameShort"="Cell_Voltage_10", "NumBits"=16, "ScaleFac"=1.0, "ScaleOff"=0.0, "StartBit"=16, "Unit"="V"}, {"ByteOrdr"=0, "Comment"="", "DataType"=1, "Default"=0.0, "Max"=5.0, "Min"=0.0, "NameShort"="Cell_Voltage_11", "NumBits"=16, "ScaleFac"=1.0, "ScaleOff"=0.0, "StartBit"=32, "Unit"="V"}, {"ByteOrdr"=0, "Comment"="", "DataType"=1, "Default"=0.0, "Max"=5.0, "Min"=0.0, "NameShort"="Cell_Voltage_12", "NumBits"=16, "ScaleFac"=1.0, "ScaleOff"=0.0, "StartBit"=48, "Unit"="V"}, {"ByteOrdr"=0, "Comment"="", "DataType"=1, "Default"=0.0, "Max"=5.0, "Min"=0.0, "NameShort"="Cell_Voltage_9", "NumBits"=16, "ScaleFac"=1.0, "ScaleOff"=0.0, "StartBit"=0, "Unit"="V"}], "XNET Frame properties"={"NameShort"="Cell_V_Set_9_12", "ID"=192, "PayldLen"=8, "CAN.TimingType"=1, "CAN.TxTime"=0.1}}, {[{"ByteOrdr"=0, "Comment"="", "DataType"=1, "Default"=0.0, "Max"=5.0, "Min"=0.0, "NameShort"="Cell_Voltage_All", "NumBits"=16, "ScaleFac"=1.0, "ScaleOff"=0.0, "StartBit"=0, "Unit"="V"}], "XNET Frame properties"={"NameShort"="Cell_V_Set_All", "ID"=1280, "PayldLen"=2, "CAN.TimingType"=1, "CAN.TxTime"=0.1}}, {[{"ByteOrdr"=0, "Comment"="", "DataType"=1, "Default"=0.0, "Max"=1.0, "Min"=0.0, "NameShort"="AI_1_4_HIL_BCast_Enable", "NumBits"=1, "ScaleFac"=1.0, "ScaleOff"=0.0, "StartBit"=9, "Unit"=""}, {"ByteOrdr"=0, "Comment"="", "DataType"=1, "Default"=0.0, "Max"=1.0, "Min"=0.0, "NameShort"="AI_5_8_HIL_BCast_Enable", "NumBits"=1, "ScaleFac"=1.0, "ScaleOff"=0.0, "StartBit"=10, "Unit"=""}, {"ByteOrdr"=0, "Comment"="", "DataType"=1, "Default"=0.0, "Max"=1.0, "Min"=0.0, "NameShort"="AO_HIL_Set_Enable", "NumBits"=1, "ScaleFac"=1.0, "ScaleOff"=0.0, "StartBit"=1, "Unit"=""}, {"ByteOrdr"=0, "Comment"="", "DataType"=1, "Default"=0.0, "Max"=1000.0, "Min"=0.0, "NameShort"="Calibration_Mode", "NumBits"=1, "ScaleFac"=1.0, "ScaleOff"=0.0, "StartBit"=16, "Unit"=""}, {"ByteOrdr"=0, "Comment"="", "DataType"=1, "Default"=0.0, "Max"=1.0, "Min"=0.0, "NameShort"="DIO_HIL_BCast_Enable", "NumBits"=1, "ScaleFac"=1.0, "ScaleOff"=0.0, "StartBit"=8, "Unit"=""}, {"ByteOrdr"=0, "Comment"="", "DataType"=1, "Default"=0.0, "Max"=1.0, "Min"=0.0, "NameShort"="DIO_HIL_Set_Enable", "NumBits"=1, "ScaleFac"=1.0, "ScaleOff"=0.0, "StartBit"=0, "Unit"=""}], "XNET Frame properties"={"NameShort"="Configure", "ID"=1024, "PayldLen"=3, "CAN.TimingType"=1, "CAN.TxTime"=0.1}}, {[{"ByteOrdr"=0, "Comment"="", "DataType"=1, "Default"=0.0, "Max"=1.0, "Min"=0.0, "NameShort"="Calibration_Enable", "NumBits"=1, "ScaleFac"=1.0, "ScaleOff"=0.0, "StartBit"=0, "Unit"=""}, {"ByteOrdr"=1, "Comment"="", "DataType"=1, "Default"=0.0, "Max"=1.0, "Min"=0.0, "NameShort"="PID_Disable", "NumBits"=1, "ScaleFac"=1.0, "ScaleOff"=0.0, "StartBit"=1, "Unit"=""}, {"ByteOrdr"=2, "Comment"="", "DataType"=1, "Default"=0.0, "Max"=1.0, "Min"=0.0, "NameShort"="Precision_Mode_Enable", "NumBits"=1, "ScaleFac"=1.0, "ScaleOff"=0.0, "StartBit"=8, "Unit"=""}], "XNET Frame properties"={"NameShort"="OperationalConfig", "ID"=1040, "PayldLen"=2, "CAN.TimingType"=1, "CAN.TxTime"=0.1}}, {[{"ByteOrdr"=0, "Comment"="", "DataType"=1, "Default"=0.0, "Max"=255.0, "Min"=0.0, "NameShort"="DIO_1_8", "NumBits"=8, "ScaleFac"=1.0, "ScaleOff"=0.0, "StartBit"=0, "Unit"=""}], "XNET Frame properties"={"NameShort"="DIO_Readback_1_8", "ID"=640, "PayldLen"=8, "CAN.TimingType"=0, "CAN.TxTime"=0.01}}, {[{"ByteOrdr"=0, "Comment"="", "DataType"=1, "Default"=0.0, "Max"=255.0, "Min"=0.0, "NameShort"="DIO_Direction", "NumBits"=8, "ScaleFac"=1.0, "ScaleOff"=0.0, "StartBit"=8, "Unit"=""}, {"ByteOrdr"=0, "Comment"="", "DataType"=1, "Default"=0.0, "Max"=255.0, "Min"=0.0, "NameShort"="DIO_Output_Val", "NumBits"=8, "ScaleFac"=1.0, "ScaleOff"=0.0, "StartBit"=0, "Unit"=""}], "XNET Frame properties"={"NameShort"="Digital_IO_Set_1_8", "ID"=512, "PayldLen"=2, "CAN.TimingType"=1, "CAN.TxTime"=0.1}}, {[{"ByteOrdr"=0, "Comment"="Set to True to enable HIL mode", "DataType"=1, "Default"=0.0, "Max"=1000.0, "Min"=0.0, "NameShort"="Enable", "NumBits"=1, "ScaleFac"=1.0, "ScaleOff"=0.0, "StartBit"=0, "Unit"=""}], "XNET Frame properties"={"NameShort"="HIL_Mode", "ID"=128, "PayldLen"=1, "CAN.TimingType"=1, "CAN.TxTime"=0.1}}, {[{"ByteOrdr"=0, "Comment"="", "DataType"=1, "Default"=0.0, "Max"=1.0, "Min"=0.0, "NameShort"="Fan_Fail_1", "NumBits"=1, "ScaleFac"=1.0, "ScaleOff"=0.0, "StartBit"=0, "Unit"=""}, {"ByteOrdr"=0, "Comment"="", "DataType"=1, "Default"=0.0, "Max"=1.0, "Min"=0.0, "NameShort"="Fan_Fail_2", "NumBits"=1, "ScaleFac"=1.0, "ScaleOff"=0.0, "StartBit"=1, "Unit"=""}, {"ByteOrdr"=0, "Comment"="", "DataType"=1, "Default"=0.0, "Max"=1.0, "Min"=0.0, "NameShort"="Fan_Fail_3", "NumBits"=1, "ScaleFac"=1.0, "ScaleOff"=0.0, "StartBit"=2, "Unit"=""}, {"ByteOrdr"=0, "Comment"="", "DataType"=1, "Default"=0.0, "Max"=1.0, "Min"=0.0, "NameShort"="Fan_Fail_4", "NumBits"=1, "ScaleFac"=1.0, "ScaleOff"=0.0, "StartBit"=3, "Unit"=""}, {"ByteOrdr"=0, "Comment"="", "DataType"=1, "Default"=0.0, "Max"=1.0, "Min"=0.0, "NameShort"="Inhibit_State", "NumBits"=1, "ScaleFac"=1.0, "ScaleOff"=0.0, "StartBit"=4, "Unit"=""}, {"ByteOrdr"=0, "Comment"="", "DataType"=1, "Default"=0.0, "Max"=1000.0, "Min"=0.0, "NameShort"="Temp_Sensor_1", "NumBits"=8, "ScaleFac"=1.0, "ScaleOff"=0.0, "StartBit"=8, "Unit"="Degrees C"}, {"ByteOrdr"=0, "Comment"="", "DataType"=1, "Default"=0.0, "Max"=1000.0, "Min"=0.0, "NameShort"="Temp_Sensor_2", "NumBits"=8, "ScaleFac"=1.0, "ScaleOff"=0.0, "StartBit"=16, "Unit"="Degrees C"}, {"ByteOrdr"=0, "Comment"="", "DataType"=1, "Default"=0.0, "Max"=1000.0, "Min"=0.0, "NameShort"="Temp_Sensor_3", "NumBits"=8, "ScaleFac"=1.0, "ScaleOff"=0.0, "StartBit"=24, "Unit"="Degrees C"}], "XNET Frame properties"={"NameShort"="System_Status", "ID"=256, "PayldLen"=8, "CAN.TimingType"=0, "CAN.TxTime"=1.0}}] {"XNET Frame properties"."ID" format="%.0x"}
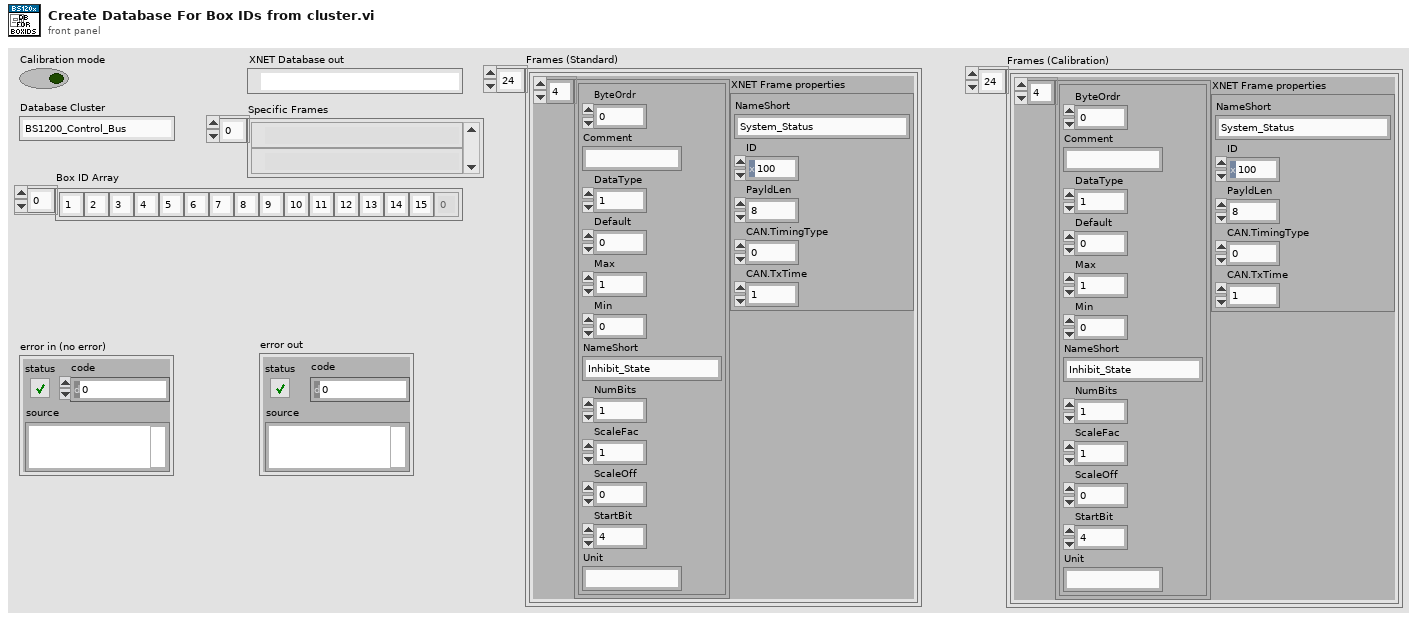
[diagram p1: front panel]
types:
  T1 = typedef "BS120x Driver.lvlib/BS120x.lvclass/XNET Signal properties.ctl" = cluster{"ByteOrdr":u32, "Comment":string, "DataType":u32, "Default":dbl, "Max":dbl, "Min":dbl, "NameShort":string, "NumBits":u32, "ScaleFac":dbl, "ScaleOff":dbl, "StartBit":u32, "Unit":string}
  T2 = typedef "BS120x Driver.lvlib/BS120x.lvclass/XNET Frame properties.ctl" = cluster{"NameShort":string, "ID":u32, "PayldLen":u32, "CAN.TimingType":u32, "CAN.TxTime":dbl}
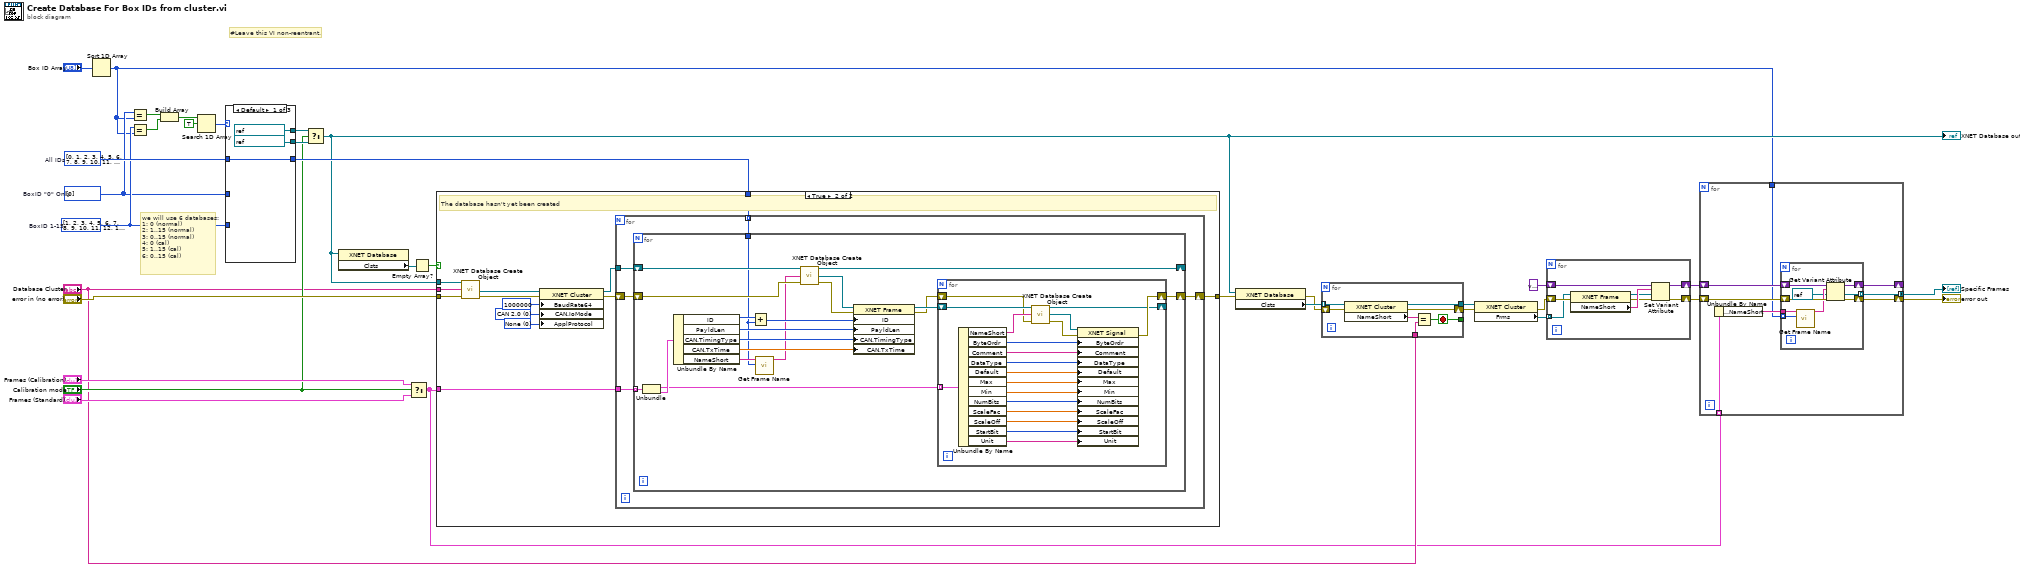
[diagram p0: block diagram]
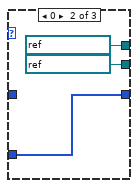
[diagram p2: hidden frame]
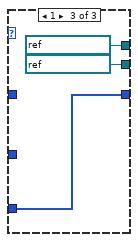
[diagram p3: hidden frame]
diagram:
  w26 = u8[] [0, 1, 2, 3, 4, 5, 6, 7, 8, 9, 10, 11, 12, 13, 14, 15]  # All IDs
  w25 = u8[] [1, 2, 3, 4, 5, 6, 7, 8, 9, 10, 11, 12, 13, 14, 15]  # BoxID 1-15
  w22 = u8[] [0]  # BoxID "0" Only
  # "#Leave this VI non-reentrant."
  # "we will use 6 databases:\n1: 0 (normal)\n2: 1..15 (normal)\n3: 0..15 (normal)\n4: 0 (cal)\n5: 1..15 (cal)\n6: 0..15 (cal)"
  n1 = Sort 1D Array(array="Box ID Array") -> (sorted array=w3:u8[])
  n2 = Equal?(x=w22, y=w3) -> (x = y?=w30:bool)
  n3 = Equal?(x=w25, y=w3) -> (x = y?=w29:bool)
  n4 = Build Array(w30, w29) -> (w28:bool[])
  n5 = Search 1D Array(1D array=w28, element=TRUE) -> (index of element=w21:i32)  [unwired: 1 in]
  n6 = case shown="Default" w21 {
    tunnel: w26 -> [w36 _ _]
    tunnel: [refnum<k21> ":memory3:" ("XNET Database out") refnum<k21> ":memory1:" ("XNET Database out") refnum<k21> ":memory2:" ("XNET Database out")] -> w19
    tunnel: w22 -> [_ w38 _]
    tunnel: w25 -> [_ _ w41]
    tunnel: [w36 w38 w41] -> w23
    tunnel: [refnum<k21> ":memory6:" ("XNET Database out") refnum<k21> ":memory4:" ("XNET Database out") refnum<k21> ":memory5:" ("XNET Database out")] -> w20
    frame Default {
    }
    frame 0 {
    }
    frame 1 {
    }
  }
  n7 = Select(t=w20, s="Calibration mode", f=w19) -> (s? t:f=w16:refnum<k21>)
  "XNET Database out" <- w16
  n8 = property class="XNET Database"(reference=w16) -> ("Clsts"=w31:refnum<k21>[])  [unwired: 1 in, 2 out]
  n9 = Select(t="Frames (Calibration)", s="Calibration mode", f="Frames (Standard)") -> (s? t:f=w5:cluster{T1[], "XNET Frame properties":T2}[])
  n10 = Empty Array?(array=w31) -> (empty?=w1:bool)
  n11 = case shown="True" w1 {
    tunnel: w23 -> [_ w57]
    tunnel: "error in (no error)" -> [w44 w56]
    tunnel: [w44 w55] -> w17
    tunnel: "Database Cluster" -> [_ w54]
    tunnel: w16 -> [_ w53]
    tunnel: w5 -> [_ w52]
    frame False {
    }
    frame True {
      w47 = u32 0 items=["None", "J1939"] ("Application Protocol")
      w48 = u32 0 items=["CAN 2.0", "CAN FD", "CAN FD+BRS"] ("CAN:I/O Mode")
      # "The database hasn't yet been created"
      n12 = call-poly <vilib>:"XNET Database Create Object.vi"("database in"=w53, "cluster name"=w54, "error in (no error)"=w56) -> ("cluster out"=w51:refnum<k21>, "error out"=w46:errorcluster)  [unwired: 10 in, 1 out]
      n13 = property class="XNET Cluster"(reference=w51, error in=w46, "BaudRate64"=u64 1000000 ("64bit Baud Rate"), "CAN.IoMode"=w48, "ApplProtocol"=w47) -> (reference out=w50:refnum<k21>, error out=w45:errorcluster)
      n14 = for {
        tunnel: w57 -> [w62] mode=indexing
        tunnel: w52 -> [w60]
        tunnel: w50 -> [w58]
        shift-right: [w61] -> w55
        shift-left: w45 -> [w59]
        n15 = for {
          shift-right: [w68] -> w61
          shift-left: w59 -> [w66]
          tunnel: w62 -> [w64]
          tunnel: w60 -> [w79] mode=indexing
          shift-right: [w69] -> _
          shift-left: w58 -> [w81]
          n16 = Unbundle(w79) -> (w72:T1[], "XNET Frame properties"=w78:T2)
          n17 = Unbundle By Name(w78) -> ("ID"=w77:u32, "PayldLen"=w76:u32, "CAN.TimingType"=w75:u32, "CAN.TxTime"=w74:dbl, "NameShort"=w65:string)
          n18 = Add(x=w77, y=w64) -> (x+y=w73:u32)
          n19 = call "Get Frame Name.vi"("Box ID"=w64, "Frame Name"=w65) -> ("Frame Name out"=w63:string)  [unwired: 9 in]
          n20 = call-poly <vilib>:"XNET Database Create Object.vi"("cluster in"=w81, "frame name"=w63, "error in (no error)"=w66) -> ("cluster out"=w69:refnum<k21>, "frame out"=w80:refnum<k21>, "error out"=w70:errorcluster)  [unwired: 10 in]
          n21 = property class="XNET Frame"(reference=w80, error in=w70, "ID"=w73, "PayldLen"=w76, "CAN.TimingType"=w75, "CAN.TxTime"=w74) -> (reference out=w71:refnum<k21>, error out=w67:errorcluster)
          n22 = for {
            shift-right: [w100] -> w68
            shift-left: w67 -> [w96]
            tunnel: w72 -> [w98] mode=indexing
            shift-right: [w83] -> _
            shift-left: w71 -> [w99]
            n23 = Unbundle By Name(w98) -> ("NameShort"=w97:string, "ByteOrdr"=w95:u32, "Comment"=w94:string, "DataType"=w93:u32, "Default"=w92:dbl, "Max"=w91:dbl, "Min"=w90:dbl, "NumBits"=w89:u32, "ScaleFac"=w88:dbl, "ScaleOff"=w87:dbl, "StartBit"=w86:u32, "Unit"=w85:string)
            n24 = call-poly <vilib>:"XNET Database Create Object.vi"("frame in"=w99, "signal name"=w97, "error in (no error)"=w96) -> ("frame out"=w83:refnum<k21>, "signal out"=w84:refnum<k21>, "error out"=w82:errorcluster)  [unwired: 10 in]
            n25 = property class="XNET Signal"(reference=w84, error in=w82, "ByteOrdr"=w95, "Comment"=w94, "DataType"=w93, "Default"=w92, "Max"=w91, "Min"=w90, "NumBits"=w89, "ScaleFac"=w88, "ScaleOff"=w87, "StartBit"=w86, "Unit"=w85) -> (error out=w100:errorcluster)  [unwired: 1 out]
          }
        }
      }
    }
  }
  n26 = property class="XNET Database"(reference=w16, error in=w17) -> (error out=w14:errorcluster, "Clsts"=w15:refnum<k21>[])  [unwired: 1 out]
  n27 = for {
    tunnel: w15 -> [w106] mode=indexing
    shift-right: [w102] -> w9
    shift-left: w14 -> [w107]
    tunnel: "Database Cluster" -> [w104]
    tunnel: [w103] -> w12
    tunnel: [w101] -> _
    stop <- w101 stop-if-true
    n28 = property class="XNET Cluster"(reference=w106, error in=w107) -> (reference out=w103:refnum<k21>, error out=w102:errorcluster, "NameShort"=w105:string)
    n29 = Equal?(x=w105, y=w104) -> (x = y?=w101:bool)
  }
  n30 = property class="XNET Cluster"(reference=w12, error in=w9) -> (error out=w8:errorcluster, "Frms"=w11:refnum<k21>[])  [unwired: 1 out]
  n31 = for {
    tunnel: w11 -> [w113] mode=indexing
    shift-right: [w109] -> w6
    shift-left: w8 -> [w114]
    shift-right: [w108] -> w7
    shift-left: variant -> [w115]
    n32 = property class="XNET Frame"(reference=w113, error in=w114) -> (reference out=w111:refnum<k21>, error out=w110:errorcluster, "NameShort"=w112:string)
    n33 = Set Variant Attribute(Variant=w115, name=w112, value=w111, error in=w110) -> (Variant out=w108:variant, error out=w109:errorcluster)  [unwired: 1 out]
  }
  n34 = for {
    shift-right: [w122] -> w2
    shift-left: w6 -> [w118]
    shift-right: [w121] -> _
    shift-left: w7 -> [w123]
    tunnel: w5 -> [w120] mode=indexing
    tunnel: [w117] -> w4 mode=concatenating
    tunnel: w3 -> [w116]
    n35 = Unbundle By Name(w120) -> ("XNET Frame properties.NameShort"=w119:string)
    n36 = for {
      tunnel: w119 -> [w129]
      tunnel: [w125] -> w117 mode=indexing
      shift-right: [w130] -> w121
      shift-left: w123 -> [w132]
      shift-right: [w131] -> w122
      shift-left: w118 -> [w128]
      tunnel: w116 -> [w124] mode=indexing
      n37 = call "Get Frame Name.vi"("Box ID"=w124, "Frame Name"=w129) -> ("Frame Name out"=w127:string)  [unwired: 9 in]
      n38 = Get Variant Attribute(Variant=w132, name=w127, default value (empty Variant)=refnum<k21> refnum ("XNET Frame"), error in=w128) -> (duplicate Variant=w130:variant, value=w125:refnum<k21>, error out=w131:errorcluster)  [unwired: 1 out]
    }
  }
  "error out" <- w2
  "Specific Frames" <- w4
